vi "CRYLogin.vi"() -> (0 "Exit?":bool, 1 "Remember?":bool, 2 "Passwords out":T1, 3 "user level out":enum16{"engr", "tech", "oper"}(ring), 4 "User Name out":string)   [LabVIEW 2013]
uses:
  CRYMainGlobal.vi
panel:
  out "Remember Out":bool
  in  "Access Level":u16(ring) caption="访问级别" items=["工程师", "技术员", "操作员"]
  in  "User Name":string caption="用户名称"
  in  "Exit":bool
  in  "Setup":bool
  in  "OK":bool
  in  "Password":string caption="密码"
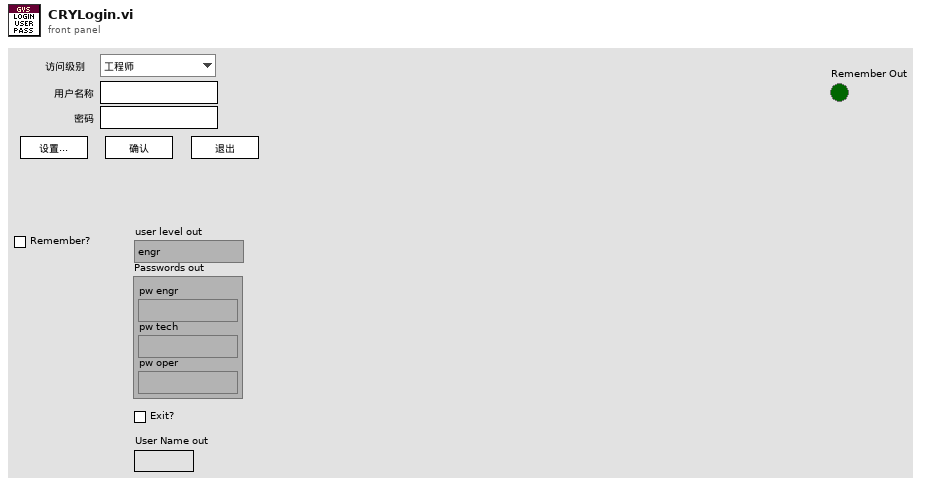
[diagram p1: front panel]
types:
  T1 = cluster{"pw engr":string, "pw tech":string, "pw oper":string}
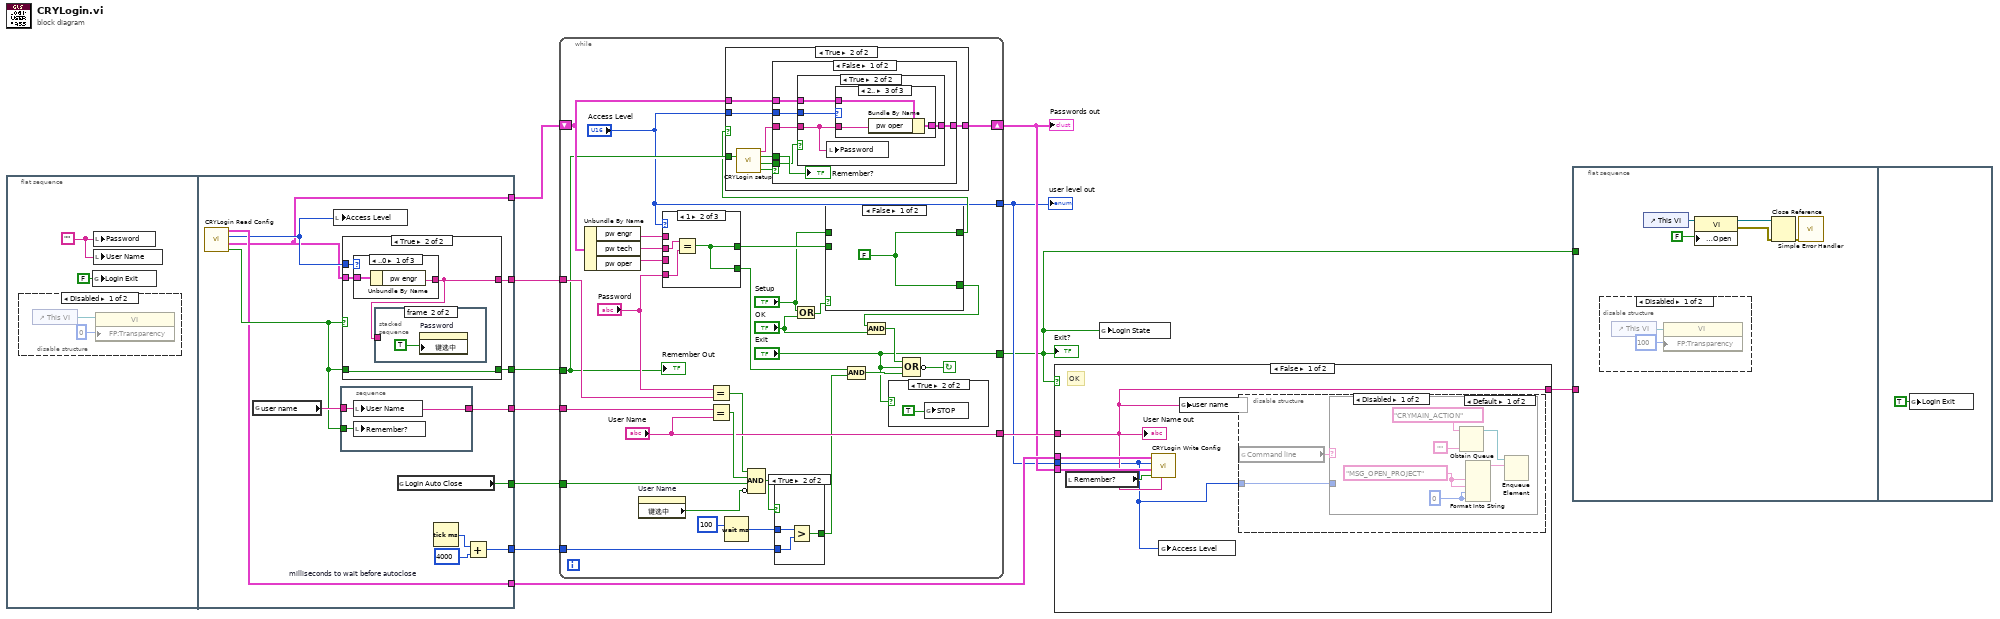
[diagram p0: block diagram]
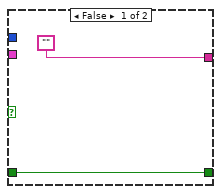
[diagram p3: hidden frame]
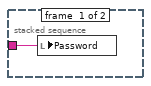
[diagram p4: hidden frame]
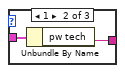
[diagram p5: hidden frame]
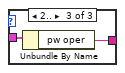
[diagram p6: hidden frame]
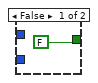
[diagram p9: hidden frame]
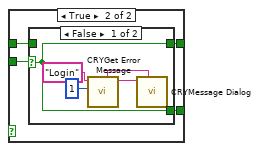
[diagram p10: hidden frame]
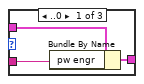
[diagram p14: hidden frame]
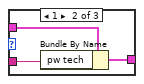
[diagram p15: hidden frame]
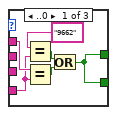
[diagram p17: hidden frame]
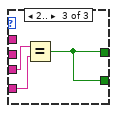
[diagram p18: hidden frame]
diagram:
  n1 = flat-sequence {
    tunnel: [w28] -> w12
    tunnel: [w27] -> w11
    tunnel: [w26] -> w10
    tunnel: [w22] -> w8
    tunnel: [w20] -> w7
    tunnel: [w17] -> w4
    tunnel: [w18] -> w2
    frame #0 {
      w14 = "" ("Password")
      n2 = disable-structure shown="Disabled" {
        frame Disabled {
          n3 = control-ref of="This VI"() -> (w16:refnum<vi>)
          n4 = property class="VI"(reference=w16, "FP:Transparency"=u8 0 ("Front Panel Window:Transparency")) -> ()  [unwired: 1 in, 2 out]
        }
        frame Enabled {
        }
      }
      n5 = global write "CRYMainGlobal.vi" "Login Exit"(FALSE ("Login Exit")) -> ()
      n6 = local write "Password"(w14) -> ()
      n7 = local write "User Name"(w14) -> ()
    }
    frame #1 {
      w24 = u32 4000  # milliseconds to wait before autoclose
      n8 = call "CRYLogin Read Config.vi"() -> ("Remember Out"=w21:bool, "Password out"=w18:T1, "Level Out"=w19:i32, "Login Section Out"=w20:cluster{"Key":string, "Value":string}[])  [unwired: 8 out]
      n9 = global read "CRYMainGlobal.vi" "user name"() -> (w23:string)
      n10 = local write "Access Level"(w19) -> ()
      n11 = stacked-sequence {
        tunnel: w23 -> [w30]
        tunnel: [w30] -> w27
        tunnel: w21 -> [w29]
        frame #0 {
          n12 = local write "User Name"(w30) -> ()
          n13 = local write "Remember?"(w29) -> ()
        }
      }
      n14 = case shown="True" w21 {
        tunnel: [w32 w34] -> w28
        tunnel: w19 -> [_ w36]
        tunnel: w18 -> [_ w35]
        tunnel: w21 -> [w32 w34]
        tunnel: ["" w33] -> w26
        frame False {
        }
        frame True {
          n15 = case shown="..0" w36 {
            tunnel: [w40 w42 w44] -> w33
            tunnel: w35 -> [w39 w41 w43]
            frame ..0 {
              n16 = Unbundle By Name(w39) -> ("pw engr"=w40:string)
            }
            frame 1 {
              n17 = Unbundle By Name(w41) -> ("pw tech"=w42:string)
            }
            frame 2.. {
              n18 = Unbundle By Name(w43) -> ("pw oper"=w44:string)
            }
          }
          n19 = stacked-sequence {
            tunnel: w33 -> [w37 _]
            frame #0 {
              n20 = local write "Password"(w37) -> ()
            }
            frame #1 {
              n21 = property on="Password" class="Str"("键选中"=TRUE ("Key Focus")) -> ()  [unwired: 2 in, 2 out]
            }
          }
        }
      }
      n22 = global read "CRYMainGlobal.vi" "Login Auto Close"() -> (w17:bool)
      n23 = Tick Count (ms)() -> (millisecond timer value=w25:u32)
      n24 = Add(x=w25, y=w24) -> (x+y=w22:u32)
    }
  }
  n25 = while {
    tunnel: ["User Name"] -> w9
    tunnel: w8 -> [w60]
    tunnel: w4 -> [w65]
    tunnel: w10 -> [w62]
    tunnel: w11 -> [w61]
    tunnel: w12 -> [w55]
    shift-left: w2 -> [w71]
    shift-right: [w72] -> w6
    tunnel: ["Exit"] -> w1
    tunnel: ["Access Level"] -> w3
    stop <- w48 continue-if-true
    n26 = Unbundle By Name(w71) -> ("pw engr"=w75:string, "pw tech"=w74:string, "pw oper"=w73:string)
    n27 = property on="User Name" class="Str"() -> ("键选中"=w52:bool)  [unwired: 2 in, 2 out]
    n28 = case shown="1" "Access Level" {
      tunnel: "Password" -> [w127 w131 w134]
      tunnel: w75 -> [w128 _ _]
      tunnel: [w123 w129 w132] -> w69
      tunnel: w74 -> [_ w130 _]
      tunnel: w73 -> [_ _ w133]
      tunnel: [w123 w129 w132] -> w56
      frame ..0 {
        n29 = Equal?(x="9662", y=w127) -> (x = y?=w125:bool)
        n30 = Equal?(x=w128, y=w127) -> (x = y?=w124:bool)
        n31 = Or(x=w125, y=w124) -> (x .or. y?=w123:bool)
      }
      frame 1 {
        n32 = Equal?(x=w130, y=w131) -> (x = y?=w129:bool)
      }
      frame 2.. {
        n33 = Equal?(x=w133, y=w134) -> (x = y?=w132:bool)
      }
    }
    n34 = Equal?(x="Password", y=w62) -> (x = y?=w45:bool)
    n35 = Equal?(x=w61, y="User Name") -> (x = y?=w64:bool)
    n36 = Wait (ms)(milliseconds to wait=u32 100) -> (millisecond timer value=w50:u32)
    n37 = Compound Arithmetic op=AND(w45, w64, w65, invert w52) -> (w59:bool)
    n38 = case shown="True" w59 {
      tunnel: w60 -> [_ w80]
      tunnel: [FALSE w79] -> w54
      tunnel: w50 -> [_ w78]
      frame False {
      }
      frame True {
        n39 = Greater?(x=w78, y=w80) -> (0:w79:bool)
      }
    }
    n40 = Or(x="Setup", y="OK") -> (x .or. y?=w67:bool)
    n41 = case shown="False" w67 {
      tunnel: [w81 w84] -> w70
      tunnel: w69 -> [_ w85]
      tunnel: [w81 w83] -> w49
      tunnel: "Setup" -> [_ w82]
      frame False {
        w81 = FALSE
      }
      frame True {
        n42 = case shown="False" w85 {
          selector: w85 -> [w90 w92]
          tunnel: [w90 w92] -> w84
          tunnel: [w90 w91] -> w83
          tunnel: w82 -> [_ w91]
          frame False {
            n43 = call "CRYGet Error Message.vi"("Error No"=1, "Kind"="Login") -> ("Message"=w87:string, "Window Title"=w86:string)  [unwired: 4 in, 4 out]
            n44 = call "CRYMessage Dialog.vi"("Window Title"=w86, "Message Content"=w87) -> ()  [unwired: 8 in, 2 out]
          }
          frame True {
          }
        }
      }
    }
    n45 = case shown="True" w49 {
      tunnel: "Access Level" -> [_ w98]
      tunnel: [w93 w97] -> w72
      tunnel: w71 -> [w93 w96]
      tunnel: w55 -> [_ w94]
      frame False {
      }
      frame True {
        n46 = call "CRYLogin setup.vi"("Ask"=w94) -> ("Cancelled?"=w101:bool, "New PW?"=w95:bool, "Remember?"=w100:bool, "Password"=w99:string)  [unwired: 3 in, 2 out]
        n47 = case shown="False" w101 {
          tunnel: w100 -> [w107 _]
          tunnel: w99 -> [w103 _]
          tunnel: w98 -> [w106 _]
          tunnel: [w105 w122] -> w97
          tunnel: w96 -> [w104 w122]
          tunnel: w95 -> [w102 _]
          frame False {
            n48 = case shown="True" w102 {
              tunnel: w103 -> [_ w110]
              tunnel: w104 -> [w108 w109]
              tunnel: [w108 w112] -> w105
              tunnel: w106 -> [_ w111]
              frame False {
              }
              frame True {
                n49 = local write "Password"(w110) -> ()
                n50 = case shown="2.." w111 {
                  tunnel: w110 -> [w114 w117 w121]
                  tunnel: [w115 w118 w120] -> w112
                  tunnel: w109 -> [w113 w116 w119]
                  frame ..0 {
                    n51 = Bundle By Name(cluster=w113, "pw engr"=w114) -> (w115:T1)
                  }
                  frame 1 {
                    n52 = Bundle By Name(cluster=w116, "pw tech"=w117) -> (w118:T1)
                  }
                  frame 2.. {
                    n53 = Bundle By Name(cluster=w119, "pw oper"=w121) -> (w120:T1)
                  }
                }
              }
            }
            "Remember?" <- w107
          }
          frame True {
          }
        }
      }
    }
    n54 = Compound Arithmetic op=AND(w56, w54) -> (w53:bool)
    n55 = And(x=w70, y="OK") -> (x .and. y?=w57:bool)
    n56 = case shown="True" "Exit" {
      frame False {
      }
      frame True {
        n57 = global write "CRYMainGlobal.vi" "STOP"(TRUE ("STOP")) -> ()
      }
    }
    n58 = Compound Arithmetic op=OR(w57, "Exit", w53) -> (invert w48:bool)
    "Remember Out" <- w55
  }
  "user level out" <- w3
  "Exit?" <- w1
  "Passwords out" <- w6
  n59 = case shown="False" w1 {
    tunnel: w9 -> [w136 w148]
    tunnel: w7 -> [w137 _]
    tunnel: w3 -> [w135 _]
    tunnel: w6 -> [w139 _]
    tunnel: [w136 w148] -> w5
    frame False {
      # "OK"
      n60 = local read "Remember?"() -> (w138:bool)
      n61 = call "CRYLogin Write Config.vi"("User Name In"=w136, "Remember In"=w138, "Password  In"=w139, "Level In"=w135, "Login Section In"=w137) -> ()  [unwired: 7 out]
      n62 = global write "CRYMainGlobal.vi" "Access Level"(w135) -> ()
      n63 = global write "CRYMainGlobal.vi" "user name"(w136) -> ()
      n64 = disable-structure shown="Disabled" {
        disable-tunnel: w135 -> [w141 _]
        frame Disabled {
          n65 = global read "CRYMainGlobal.vi" "Command line"() -> (w140:string)
          n66 = case shown="Default" w140 {
            tunnel: w141 -> [_ _]
            frame Default {
              w142 = 0 ("input 3")
              w147 = "MSG_OPEN_PROJECT" ("input 1")
              n67 = Obtain Queue(name (unnamed)="CRYMAIN_ACTION" ("YAxisTitle"), element data type="" ("Action Type")) -> (queue out=w146:refnum<queue>)  [unwired: 3 in, 2 out]
              n68 = Format Into String(w147, w147, w142, w142) -> (resulting string=w145:string)  [unwired: 3 in, 1 out]
              n69 = Enqueue Element(queue=w146, element=w145) -> ()  [unwired: 1 in, 4 out]
            }
            frame "" {
            }
          }
        }
        frame Enabled {
        }
      }
      "User Name out" <- w136
    }
    frame True {
      # "Exit"
    }
  }
  n70 = global write "CRYMainGlobal.vi" "Login State"(w1) -> ()
  n71 = flat-sequence {
    tunnel: w5 -> [_]
    tunnel: w1 -> [_]
    frame #0 {
      n72 = disable-structure shown="Disabled" {
        frame Disabled {
          n73 = control-ref of="This VI"() -> (w155:refnum<vi>)
          n74 = property class="VI"(reference=w155, "FP:Transparency"=u8 100 ("Front Panel Window:Transparency")) -> ()  [unwired: 1 in, 2 out]
        }
        frame Enabled {
        }
      }
      n75 = control-ref of="This VI"() -> (w153:refnum<vi>)
      n76 = property class="VI"(reference=w153, "Front Panel Window:Open"=FALSE ("Front Panel.Open")) -> (reference out=w151:refnum<vi>, error out=w150:errorcluster)  [unwired: 1 in]
      n77 = Close Reference(reference=w151, error in (no error)=w150) -> (error out=w149:errorcluster)
      n78 = call <vilib>:"Simple Error Handler.vi"("error in (no error)"=w149) -> ()  [unwired: 2 in, 7 out]
    }
    frame #1 {
      n79 = global write "CRYMainGlobal.vi" "Login Exit"(TRUE ("Login Exit")) -> ()
    }
  }
